vi "Popup Debug Message Box.vi"(0 "code":i32, 5 "Message":string) -> ()   [LabVIEW 2013, in "AIT 664 Custom Device.lvlib"]
doc: "Message box to display a popup while debugging"
uses:
  AIT 664 Custom Device.lvlib
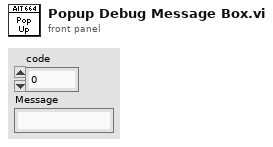
[diagram p1: front panel]
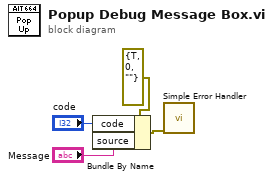
[diagram p0: block diagram]
diagram:
  n1 = Bundle By Name(cluster=errorcluster {"status"=TRUE, "code"=0, "source"=""} ("error constant"), "code"="code", "source"="Message") -> (w4:errorcluster)
  n2 = call <vilib>:"Simple Error Handler.vi"("error in (no error)"=w4) -> ()  [unwired: 4 in, 5 out]
